vi "Assert Equal Variant.vi"(6 "error code (1)":i32=1, 7 "message":string, 8 "error in (no error)":errorcluster, 10 "Y":variant, 11 "X":variant) -> (0 "error out":errorcluster)   [LabVIEW 2009]
uses:
  lvlib/Pink Elephant/Pink Elephant.lvlib
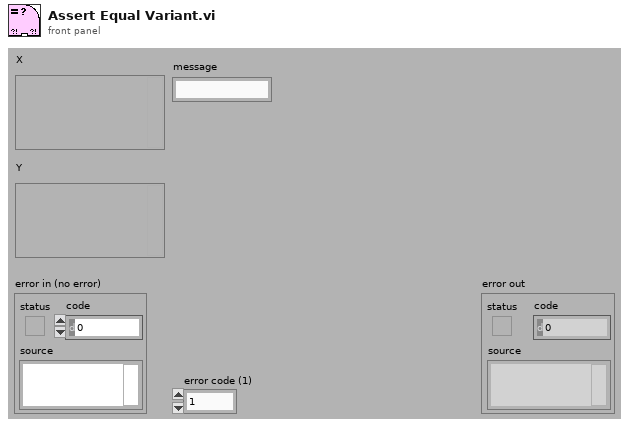
[diagram p1: front panel]
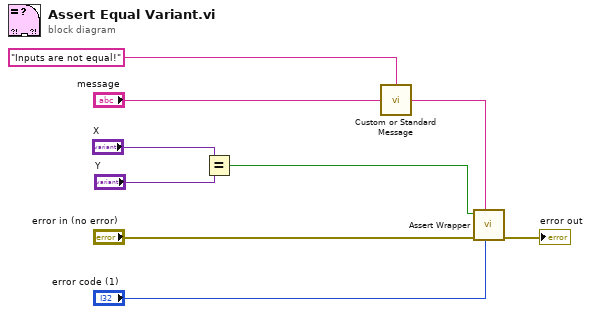
[diagram p0: block diagram]
diagram:
  n1 = Equal?(x="X", y="Y") -> (x = y?=w1:bool)
  n2 = call "Custom or Standard Message.vi"("Custom Message"="message", "Standard Message"="Inputs are not equal!") -> ("Message"=w5:string)
  n3 = call "Assert Wrapper.vi"("error code (1)"="error code (1)", "Message"=w5, "error in (no error)"="error in (no error)", "Assert?"=w1) -> ("error out"=→"error out":errorcluster)  [unwired: 7 in]
